vi "读取-删除文件.vi"(8 "错误输入":errorcluster) -> (0 "error out":errorcluster caption="错误输出", 3 "文本":string[](array[string]))   [LabVIEW 2016, in "数据传输系统-05.lvlib"]
uses:
  <vilib>/Utility/sysdir.llb/System Directory Type.ctl
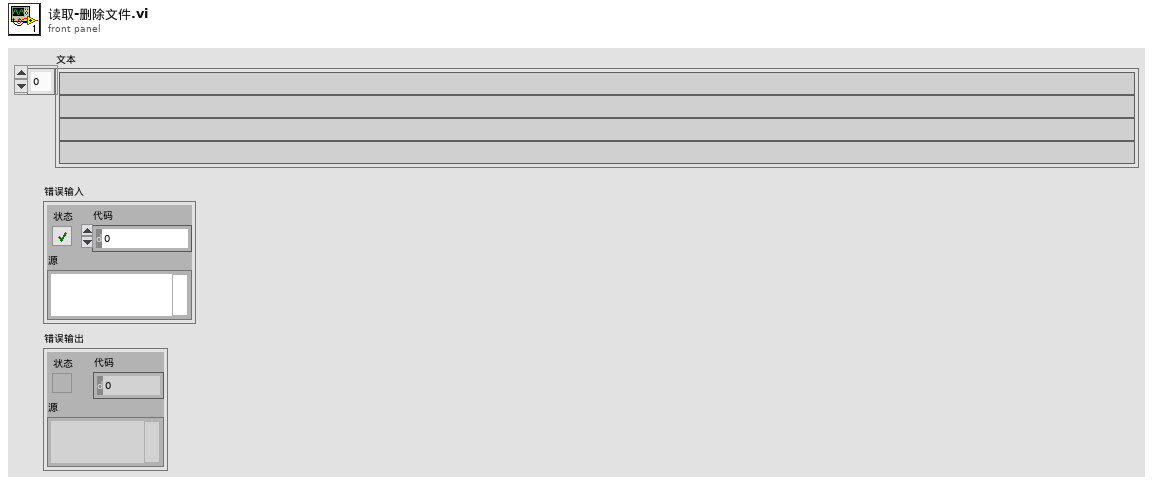
[diagram p1: front panel]
types:
  T1 = typedef "System Directory Type.ctl" = i32
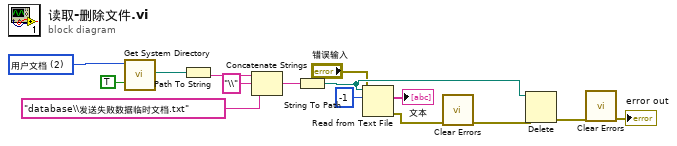
[diagram p0: block diagram]
diagram:
  w10 = T1 2 items=["用户目录"=0, "用户桌面"=1, "用户文档"=2, "用户应用程序数据"=3, "用户设置"=4, "用户临时目录"=5, "公共文档"=6, "公共应用程序数据"=7, "公共设置"=8, "公共缓存"=13, "系统核心库"=9, "系统安装库"=10, "应用程序文件"=11, "启动盘根目录"=12] ("system directory type")
  n1 = call <vilib>:"Get System Directory.vi"("create directory if not found? (F)"=TRUE, "system directory type"=w10) -> ("system directory"=w8:path)  [unwired: 9 in]
  n2 = Path To String(path=w8) -> (string=w12:string)
  n3 = Concatenate Strings(w12, "\\" ("字符串"), "database\\发送失败数据临时文档.txt" ("字符串")) -> (w15:string)
  n4 = String To Path(string=w15) -> (path=w7:path)
  n5 = Read from Text File(file (use dialog)=w7, count=-1 ("计数"), error in="错误输入") -> (text=→"文本":string[], error out=w6:errorcluster)  [unwired: 1 in, 2 out]
  n6 = call <vilib>:"Clear Errors.vi"("error in (no error)"=w6) -> ("error out"=w5:errorcluster)  [unwired: 5 in, 1 out]
  n7 = Delete(path (use dialog)=w7, error in=w5) -> (error out=w4:errorcluster)  [unwired: 3 in, 2 out]
  n8 = call <vilib>:"Clear Errors.vi"("error in (no error)"=w4) -> ("error out"=→"error out":errorcluster)  [unwired: 5 in, 1 out]
